vi "BinConditioning.vi"(8 "error in (no error)":errorcluster, 10 "Lower Bounds":dbl[](array[numeric]), 11 "Upper Bounds":dbl[](array[numeric])) -> (0 "error out":errorcluster, 1 "Upper Bounds":dbl[](array[numeric]), 2 "Lower Bounds":dbl[](array[numeric]), 3 "Bin Counts":i32[](array[numeric]))   [LabVIEW 2012, in "Histogram Custom Device.lvlib"]
uses:
  Histogram Custom Device.lvlib
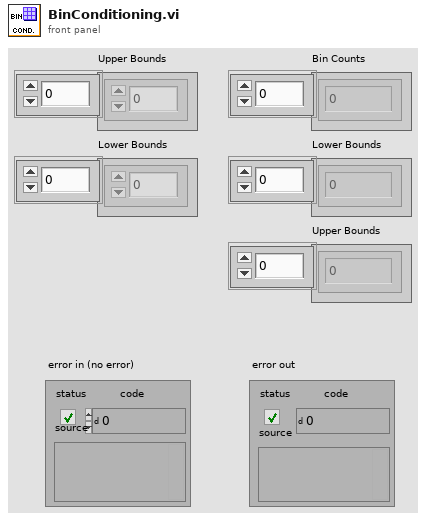
[diagram p1: front panel]
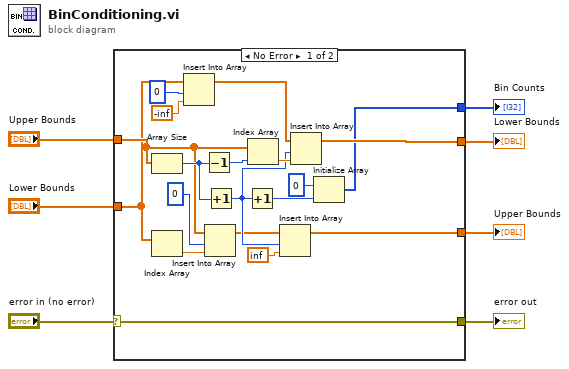
[diagram p0: block diagram]
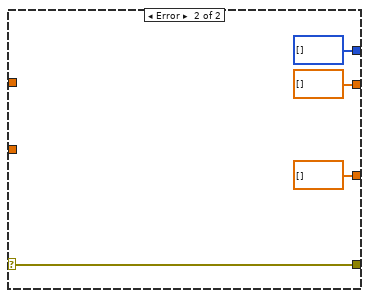
[diagram p2: hidden frame]
diagram:
  n1 = case shown="No Error" "error in (no error)" {
    selector: "error in (no error)" -> [w8 w30]
    tunnel: [w25 dbl[] [] ("Lower Bounds")] -> w7
    tunnel: "Upper Bounds" -> [w22 _]
    tunnel: "Lower Bounds" -> [w17 _]
    tunnel: [w16 dbl[] [] ("Upper Bounds")] -> w4
    tunnel: [w10 i32[] []] -> w3
    tunnel: [w8 w30] -> w1
    frame No Error {
      n2 = Array Size(array=w22) -> (size(s)=w23:i32)
      n3 = Index Array(array=w17) -> (element=w11:dbl)  [unwired: 1 in]
      n4 = Insert Into Array(array=w17, index=0, new element=-inf) -> (w20:dbl[])
      n5 = Decrement(x=w23) -> (x-1=w26:i32)
      n6 = Insert Into Array(array=w22, index=0, new element=w11) -> (w12:dbl[])
      n7 = Increment(x=w23) -> (x+1=w21:i32)
      n8 = Increment(x=w21) -> (x+1=w13:i32)
      n9 = Index Array(array=w22, index=w26) -> (element=w24:dbl)
      n10 = Insert Into Array(array=w12, index=w21, new element=inf) -> (w16:dbl[])
      n11 = Insert Into Array(array=w20, index=w21, new element=w24) -> (w25:dbl[])
      n12 = Initialize Array(0 ("element"), w13) -> (w10:i32[])
    }
    frame Error {
    }
  }
  "Lower Bounds" <- w7
  "Upper Bounds" <- w4
  "Bin Counts" <- w3
  "error out" <- w1
